vi "FTW-ZMQ-LibraryFilepath.vi"(8 "error in":errorcluster, 10 "Rediscover library?":bool) -> (0 "error out":errorcluster, 1 "ØMQ Version":string, 2 "FTW-ZMQ Library Filepath":path)   [LabVIEW 2012, in "FTW-Endpoint-ZMQ.lvclass"]
uses:
  FTW-Endpoint-ZMQ.lvclass
panel:
  # "Inputs"
  # "Outputs"
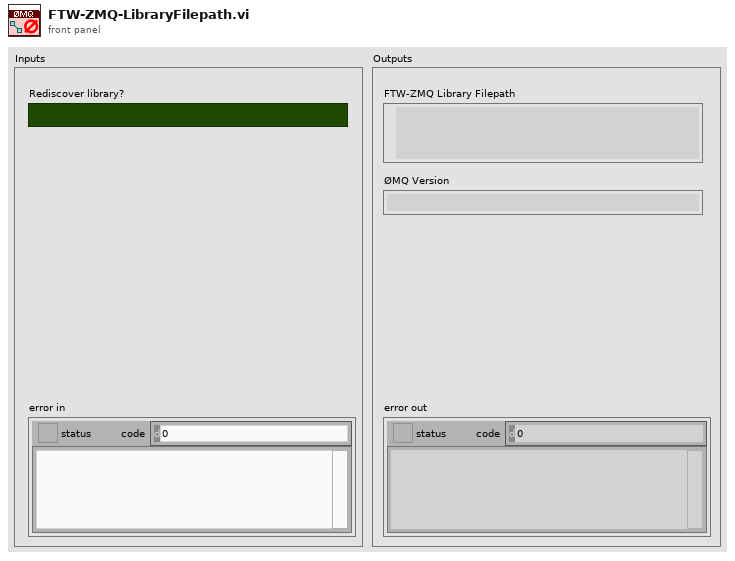
[diagram p1: front panel]
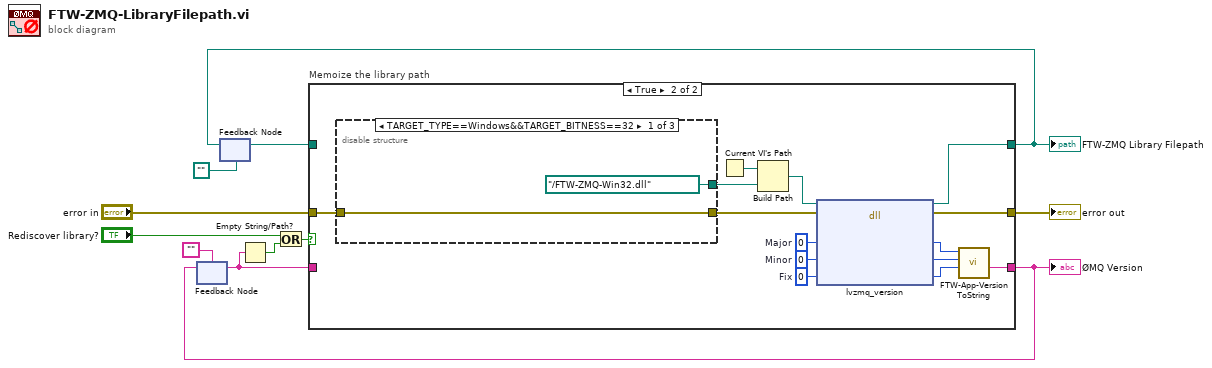
[diagram p0: block diagram]
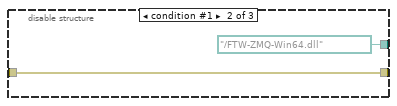
[diagram p3: hidden frame]
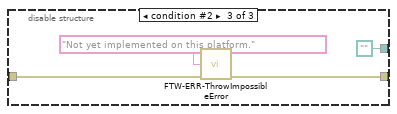
[diagram p4: hidden frame]
diagram:
  n1 = feedback #1("") -> (w4:string)
  n2 = feedback #2(path "") -> (w9:path)
  n3 = Empty String/Path?(string/path=w4) -> (empty?=w3:bool)
  n4 = Or(x="Rediscover library?", y=w3) -> (x .or. y?=w5:bool)
  n5 = case "Memoize the library path" shown="True" w5 {
    tunnel: [w14 w28] -> w8
    tunnel: "error in" -> [w13 w27]
    tunnel: [w12 w26] -> w7
    tunnel: [w13 w15] -> w10
    tunnel: w9 -> [w14 _]
    tunnel: w4 -> [w12 _]
    frame False {
    }
    frame True {
      w19 = 0  # Fix
      w20 = 0  # Minor
      w21 = 0  # Major
      n6 = disable-structure shown="TARGET_TYPE==Windows&&TARGET_BITNESS==32" {
        disable-tunnel: [path "../FTW-ZMQ-Win32.dll" path "../FTW-ZMQ-Win64.dll" path ""] -> w24
        disable-tunnel: [w30 w31 w35] -> w22
        disable-tunnel: w27 -> [w30 w31 w36]
        frame condition #0 (active) {
        }
        frame condition #1 {
        }
        frame condition #2 {
          n7 = call "FTW-ERR-ThrowImpossibleError.vi"("Reason this error should never happen"="Not yet implemented on this platform.", "error in"=w36) -> ("error out"=w35:errorcluster)  [unwired: 13 in]
        }
      }
      n8 = Current VI's Path() -> (path=w25:path)
      n9 = Build Path(base path=w25, name or relative path=w24) -> (appended path=w23:path)
      n10 = dll-call lib="?" fn="lvzmq_version" ("zmq_labview.dll:lvzmq_socket")(path in=w23, error in=w22, "Major"=w21, "Minor"=w20, "Fix"=w19) -> (path out=w28:path, error out=w15:errorcluster, "Major"=w18:i32, "Minor"=w17:i32, "Fix"=w16:i32)  [unwired: 2 in]
      n11 = call "FTW-App-VersionToString.vi"("Fix"=w16, "Minor"=w17, "Major"=w18) -> ("Version (minus Build)"=w26:string)  [unwired: 7 in, 1 out]
    }
  }
  "error out" <- w10
  "FTW-ZMQ Library Filepath" <- w8
  "ØMQ Version" <- w7
  n12 = feedback-in #1(w7) -> ()
  n13 = feedback-in #2(w8) -> ()
